vi "ziLoadSettings.vi"(3 "Error in":errorcluster, 4 "Path":string, 5 "File path (dialog if empty)":path, 6 "Handle in":T1 {"Handle" format="0x%08x"; "Conn" format="0x%08x"}) -> (0 "Error out":errorcluster, 2 "Handle out":T1 {"Handle" format="0x%08x"; "Conn" format="0x%08x"})   [LabVIEW 2015, in "Zurich Instruments LabOne.lvlib"]
uses:
  Zurich Instruments LabOne.lvlib
  ziTypeHandle.ctl
panel:
  out "lastPGAIN":dbl
  out "node_values":dbl[](array[numeric])
  out "node_paths":string[](array[string])
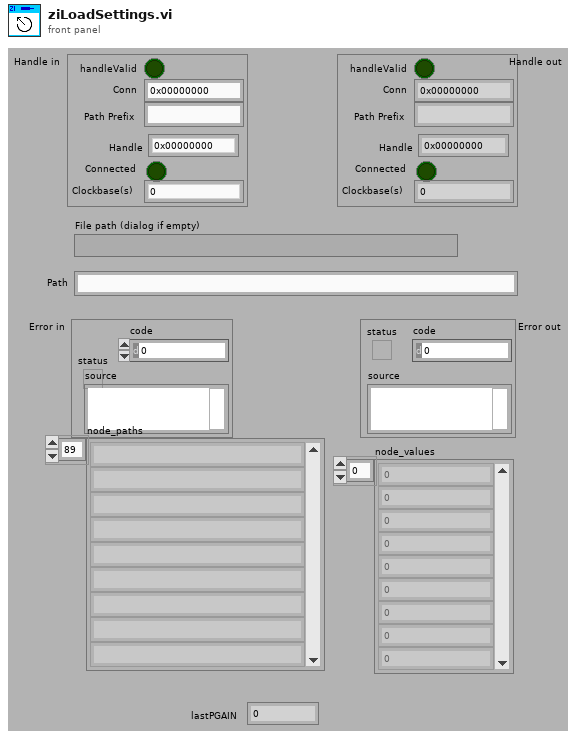
[diagram p1: front panel]
types:
  T1 = typedef "Zurich Instruments LabOne.lvlib/ziTypeHandle.ctl" = cluster{"handleValid":bool, "Conn":u64, "Path Prefix":string, "Handle":u64, "Connected":bool, "Clockbase(s)":dbl}
  T2 = enum16{"open", "replace", "create", "open or create", "replace or create", "replace or create with confirmation"}
  T3 = cluster{"Recursive":bool, "Absolut":bool, "Leafs Only":bool, "Settings Only":bool}
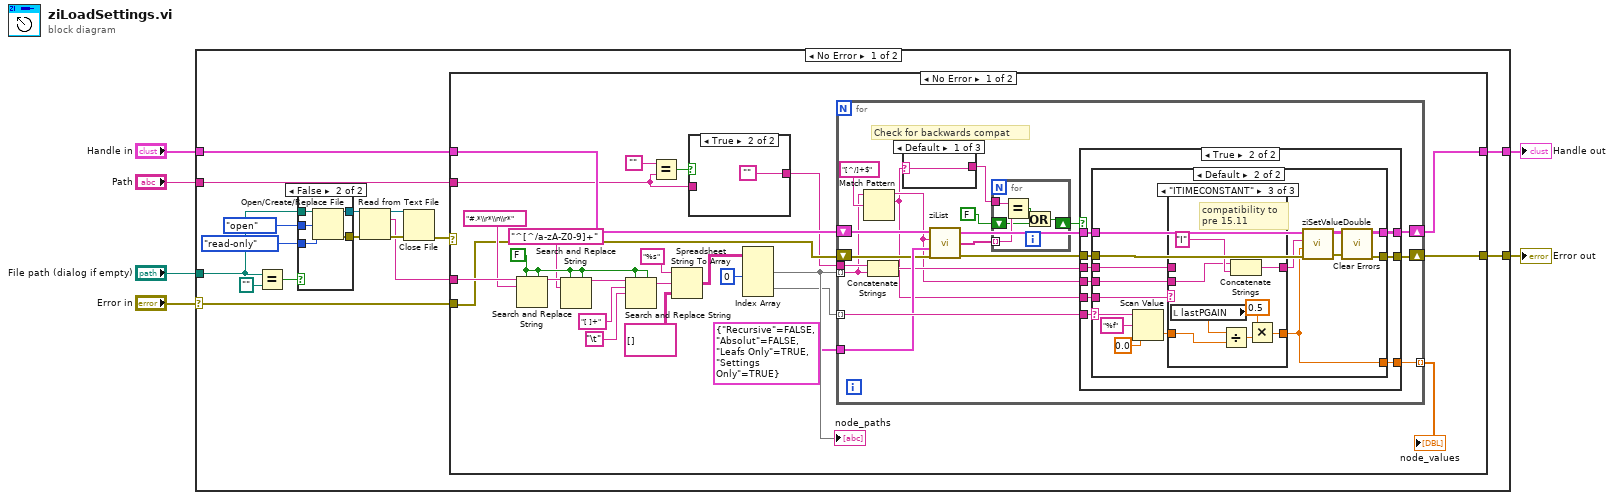
[diagram p0: block diagram]
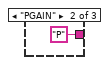
[diagram p2: hidden frame]
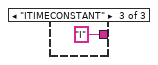
[diagram p3: hidden frame]
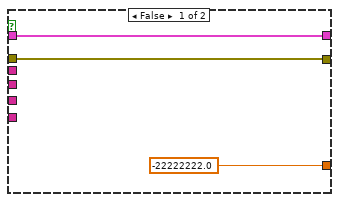
[diagram p4: hidden frame]
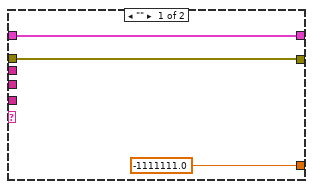
[diagram p5: hidden frame]
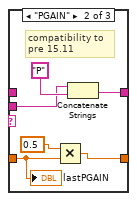
[diagram p7: hidden frame]
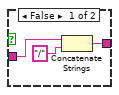
[diagram p8: hidden frame]
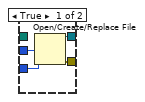
[diagram p10: hidden frame]
diagram:
  n1 = case shown="No Error" "Error in" {
    selector: "Error in" -> [w7 w135]
    tunnel: [w22 w135] -> w6
    tunnel: [w21 w136] -> w5
    tunnel: "Handle in" -> [w20 w136]
    tunnel: "File path (dialog if empty)" -> [w11 _]
    tunnel: "Path" -> [w12 _]
    frame No Error {
      n2 = Equal?(x=w11, y=path "") -> (x = y?=w10:bool)
      n3 = case shown="False" w10 {
        tunnel: T2."open" ("operation (0:open)") -> [w129 w134]
        tunnel: enum16{"read/write", "read-only", "write-only"}."read-only" ("access (0:read/write)") -> [w128 w133]
        tunnel: [w127 w132] -> w17
        tunnel: [w126 w131] -> w16
        tunnel: w11 -> [_ w130]
        frame True {
          n4 = Open/Create/Replace File(operation (0:open)=w129, access (0:read/write)=w128) -> (refnum out=w126:refnum<file>, error out=w127:errorcluster)  [unwired: 4 in, 1 out]
        }
        frame False {
          n5 = Open/Create/Replace File(file path (use dialog)=w130, operation (0:open)=w134, access (0:read/write)=w133) -> (refnum out=w131:refnum<file>, error out=w132:errorcluster)  [unwired: 3 in, 1 out]
        }
      }
      n6 = Read from Text File(file (use dialog)=w16, error in=w17) -> (refnum out=w15:refnum<file>, text=w13:string, error out=w14:errorcluster)  [unwired: 2 in, 1 out]
      n7 = Close File(refnum=w15, error in=w14) -> (error out=w8:errorcluster)  [unwired: 1 out]
      n8 = case shown="No Error" w8 {
        tunnel: [w46 w125] -> w22
        tunnel: [w45 w124] -> w21
        tunnel: w20 -> [w43 w124]
        tunnel: w13 -> [w42 _]
        tunnel: w7 -> [w30 w125]
        tunnel: w12 -> [w26 _]
        frame No Error {
          w35 = FALSE ("replace all? (F)")
          n9 = Search and Replace String(replace all?=w35, multiline?=w35, input string=w42, search string="#.*\\r*\\n\\r*") -> (result string=w41:string)  [unwired: 4 in, 3 out]
          n10 = Search and Replace String(replace all?=w35, multiline?=w35, input string=w41, search string="^[^/a-zA-Z0-9]+") -> (result string=w36:string)  [unwired: 4 in, 3 out]
          n11 = Search and Replace String(replace all?=w35, multiline?=w35, input string=w36, search string="[ ]+", replace string="\t") -> (result string=w34:string)  [unwired: 3 in, 3 out]
          n12 = Equal?(x="", y=w26) -> (x = y?=w28:bool)
          n13 = Spreadsheet String To Array(format string="%s", spreadsheet string=w34, array type (2D Dbl)=string[][] []) -> (array=w39:string[][])  [unwired: 1 in]
          n14 = case shown="True" w28 {
            tunnel: [w120 ""] -> w27
            tunnel: w26 -> [w122 _]
            frame False {
              n15 = Concatenate Strings(w122, "/" ("string")) -> (w120:string)
            }
            frame True {
            }
          }
          n16 = Index Array(array=w39, index (col) #1=0 ("disabled index (col)")) -> (element #1=w44:string[], element #2=w25:string[])  [unwired: 3 in]
          "node_paths" <- w44
          n17 = for {
            tunnel: w44 -> [w52] mode=indexing
            shift-right: [w66] -> w45
            shift-left: w43 -> [w62]
            shift-right: [w65] -> w46
            shift-left: w30 -> [w58]
            tunnel: w27 -> [w53]
            tunnel: w25 -> [w63] mode=indexing
            tunnel: [w64] -> w24 mode=indexing
            tunnel: T3 {"Recursive"=FALSE, "Absolut"=FALSE, "Leafs Only"=TRUE, "Settings Only"=TRUE} ("Flags (None)") -> [w60]
            # "Check for backwards compat"
            n18 = Match Pattern(string=w52, regular expression="[^/]+$") -> (before substring=w50:string, match substring=w49:string)  [unwired: 1 in, 2 out]
            n19 = Concatenate Strings(w53, w52) -> (w51:string)
            n20 = case shown="Default" w49 {
              selector: w49 -> [w67 _ _]
              tunnel: [w67 "P" "I"] -> w48
              frame Default {
              }
              frame "PGAIN" {
              }
              frame "ITIMECONSTANT" {
              }
            }
            n21 = call "ziList.vi"("Error In"=w58, "Flags (None)"=w60, "Path (\"\")"=w50, "Handle In"=w62) -> ("Error Out"=w59:errorcluster, "Nodes"=w56:string[], "Handle Out"=w61:T1)
            n22 = for {
              tunnel: w56 -> [w73] mode=indexing
              tunnel: w48 -> [w74]
              shift-right: [w71] -> w55
              shift-left: FALSE -> [w70]
              n23 = Equal?(x=w74, y=w73) -> (x = y?=w72:bool)
              n24 = Or(x=w72, y=w70) -> (x .or. y?=w71:bool)
            }
            n25 = case shown="True" w55 {
              tunnel: w61 -> [w77 w86]
              tunnel: w59 -> [w76 w85]
              tunnel: [w77 w84] -> w66
              tunnel: [w76 w83] -> w65
              tunnel: w51 -> [_ w82]
              tunnel: [-22222222.0 ("default (0 dbl)") w81] -> w64
              tunnel: w63 -> [_ w80]
              tunnel: w49 -> [_ w79]
              tunnel: w50 -> [_ w78]
              frame False {
              }
              frame True {
                n26 = case shown="Default" w80 {
                  selector: w80 -> [_ w96]
                  tunnel: w86 -> [w89 w103]
                  tunnel: w85 -> [w88 w102]
                  tunnel: [w89 w101] -> w84
                  tunnel: [w88 w99] -> w83
                  tunnel: w82 -> [_ w93]
                  tunnel: [-1111111.0 ("default (0 dbl)") w94] -> w81
                  tunnel: w79 -> [_ w90]
                  tunnel: w78 -> [_ w91]
                  frame "" {
                  }
                  frame Default {
                    n27 = Scan Value(string=w96, format string="%f", default (0 dbl)=0.0) -> (value=w95:dbl)  [unwired: 1 out]
                    n28 = case shown="\"ITIMECONSTANT\"" w90 {
                      tunnel: w95 -> [w105 w110 w118]
                      tunnel: [w105 w111 w117] -> w94
                      tunnel: w93 -> [w104 _ _]
                      tunnel: [w104 w106 w114] -> w92
                      tunnel: w91 -> [_ w107 w112]
                      frame Default {
                      }
                      frame "PGAIN" {
                        # "compatibility to \npre 15.11"
                        n29 = Multiply(x=0.5, y=w110) -> (x*y=w111:dbl)
                        n30 = Concatenate Strings(w107, "P" ("name or relative path")) -> (w106:string)
                        "lastPGAIN" <- w110
                      }
                      frame "ITIMECONSTANT" {
                        # "compatibility to \npre 15.11"
                        n31 = local read "lastPGAIN"() -> (w115:dbl)
                        n32 = Divide(x=w115, y=w118) -> (x/y=w119:dbl)
                        n33 = Concatenate Strings(w112, "I" ("name or relative path")) -> (w114:string)
                        n34 = Multiply(x=0.5, y=w119) -> (x*y=w117:dbl)
                      }
                    }
                    n35 = call "ziSetValueDouble.vi"("Error In"=w102, "Value"=w94, "Path"=w92, "Handle In"=w103) -> ("Error Out"=w100:errorcluster, "Handle Out"=w101:T1)  [unwired: 1 out]
                    n36 = call <vilib>:"Clear Errors.vi"("error in (no error)"=w100) -> ("error out"=w99:errorcluster)  [unwired: 5 in, 1 out]
                  }
                }
              }
            }
          }
          "node_values" <- w24
        }
        frame Error {
        }
      }
    }
    frame Error {
    }
  }
  "Handle out" <- w5
  "Error out" <- w6
